vi "Create Lookup Table Envelope Waveform.vi"(0 "Reference Waveform":T2 {"Runtime Scaling" format="%#_6p"; "Sample Rate" format="%#_6p"; "Burst Length (s)" format="%#_6p"; "PAPR (dB)" format="%.2f"; "Signal Bandwidth (Hz)" format="%#_6p"}, 5 "Lookup Table Configuration":T1={"DUT Average Input Power (dBm)"=0.0, "DUT Input Power (dBm)"=array[1024 elements], "Supply Voltage (V)"=array[1024 elements]}, 11 "error in (no error)":errorcluster) -> (4 "Lookup Table Envelope Waveform":T2 {"Runtime Scaling" format="%#_6p"; "Sample Rate" format="%#_6p"; "Burst Length (s)" format="%#_6p"; "PAPR (dB)" format="%.2f"; "Signal Bandwidth (Hz)" format="%#_6p"}, 15 "error out":errorcluster)   [LabVIEW 2019, in "Envelope Tracking.lvlib"]
doc: "Creates an envelope waveform utilizing the lookup table method."
uses:
  Envelope Tracking.lvlib
  Common/Waveform.ctl
  Typedefs/Lookup Table Configuration.ctl
  <vilib>/gmath/NI_Gmath.lvlib
  Common/Common.lvlib
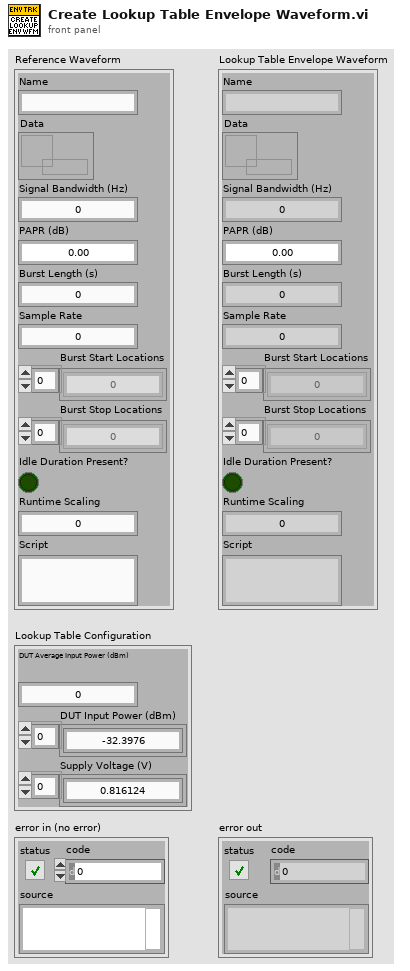
[diagram p1: front panel]
types:
  T1 = typedef "Envelope Tracking.lvlib/Lookup Table Configuration.ctl" = cluster{"DUT Average Input Power (dBm)":dbl, "DUT Input Power (dBm)":sgl[], "Supply Voltage (V)":sgl[]}
  T2 = typedef "Common.lvlib/Waveform.ctl" = cluster{"Name":string, "Data":refnum<data-value>, "Signal Bandwidth (Hz)":dbl, "PAPR (dB)":dbl, "Burst Length (s)":dbl, "Sample Rate":dbl, "Burst Start Locations":i32[], "Burst Stop Locations":i32[], "Idle Duration Present?":bool, "Runtime Scaling":dbl, "Script":string}
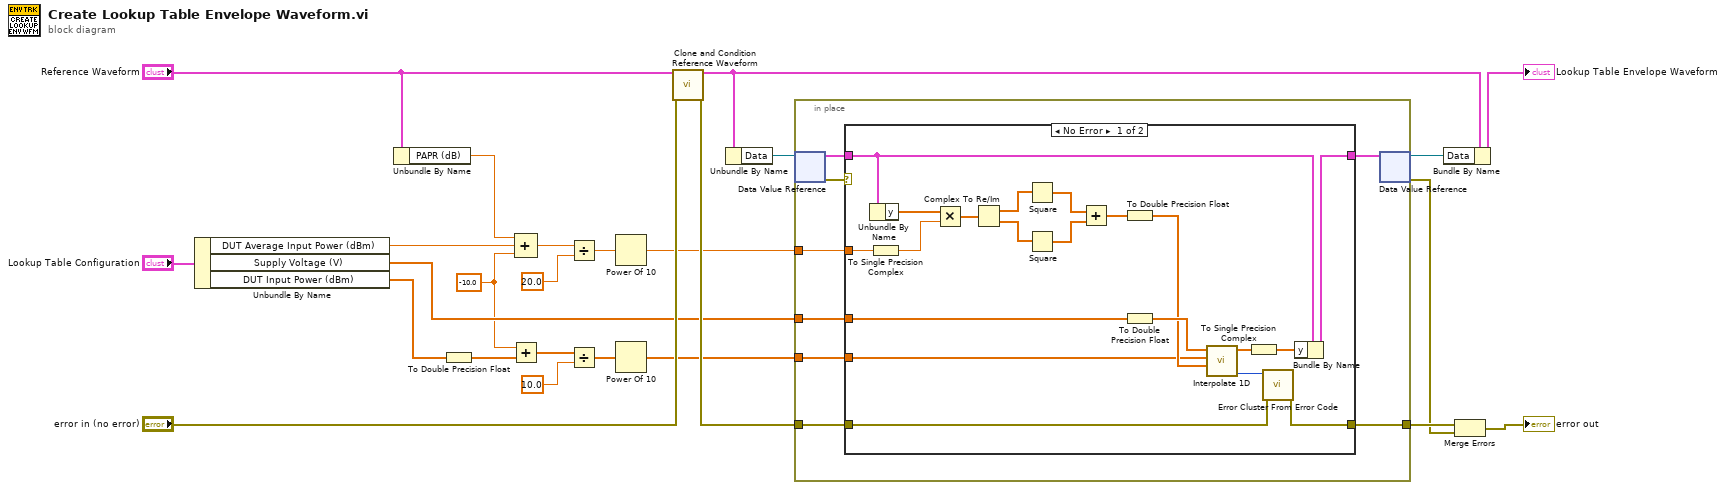
[diagram p0: block diagram]
diagram:
  w12 = -10.0 ("value")
  n1 = Unbundle By Name("Lookup Table Configuration") -> ("DUT Average Input Power (dBm)"=w19:dbl, "Supply Voltage (V)"=w14:sgl[], "DUT Input Power (dBm)"=w13:sgl[])
  n2 = Unbundle By Name("Reference Waveform") -> ("PAPR (dB)"=w1:dbl)
  n3 = To Double Precision Float(number=w13) -> (double precision float=w11:dbl[])
  n4 = Add(x=w12, y=w11) -> (x+y=w10:dbl[])
  n5 = Compound Arithmetic op=ADD(w1, w19, w12) -> (w18:dbl)
  n6 = Divide(x=w18, y=20.0) -> (x/y=w16:dbl)
  n7 = Divide(x=w10, y=10.0) -> (x/y=w8:dbl[])
  n8 = Power Of 10(x=w16) -> (10^x=w15:dbl)
  n9 = Power Of 10(x=w8) -> (10^x=w7:dbl[])
  n10 = call "Clone and Condition Reference Waveform.vi"("Reference Waveform"="Reference Waveform", "error in (no error)"="error in (no error)") -> ("Conditioned Reference Waveform"=w5:T2, "error out"=w24:errorcluster)  [unwired: 12 in]
  n11 = Unbundle By Name(w5) -> ("Data"=w4:refnum<data-value>)
  n12 = in-place {
    in-place-border: [w32] -> w23
    in-place-border: w15 -> [w30]
    in-place-border: w14 -> [w29]
    in-place-border: w7 -> [w28]
    in-place-border: w24 -> [w33]
    n13 = in-place-dvr #1(w4) -> (w27:cluster{"t0":dbl, "dt":dbl, "y":csg[]}, w31:errorcluster)
    n14 = case shown="No Error" w31 {
      tunnel: w30 -> [w51 _]
      tunnel: w29 -> [w43 _]
      tunnel: w28 -> [w39 _]
      tunnel: w27 -> [w35 w54]
      tunnel: w33 -> [w53 w55]
      tunnel: [w34 w54] -> w26
      tunnel: [w52 w55] -> w32
      frame No Error {
        n15 = Unbundle By Name(w35) -> ("y"=w49:csg[])
        n16 = To Single Precision Complex(1:w51) -> (0:w50:csg)
        n17 = Multiply(x=w49, y=w50) -> (x*y=w48:csg[])
        n18 = Complex To Re/Im(x + iy=w48) -> (x=w47:sgl[], y=w46:sgl[])
        n19 = Square(x=w47) -> (x^2=w45:sgl[])
        n20 = Square(x=w46) -> (x^2=w44:sgl[])
        n21 = Add(x=w45, y=w44) -> (x+y=w41:sgl[])
        n22 = To Double Precision Float(number=w41) -> (double precision float=w40:dbl[])
        n23 = To Double Precision Float(number=w43) -> (double precision float=w42:dbl[])
        n24 = call <vilib>:"Interpolate 1D.vi"("xi"=w40, "X"=w39, "Y"=w42) -> ("error"=w38:i32, "yi"=w37:dbl[])  [unwired: 6 in, 1 out]
        n25 = To Single Precision Complex(1:w37) -> (0:w36:csg[])
        n26 = call <vilib>:"Error Cluster From Error Code.vi"("error in (no error)"=w53, "error code (0)"=w38) -> ("error out"=w52:errorcluster)  [unwired: 7 in]
        n27 = Bundle By Name(cluster=w35, "y"=w36) -> (w34:cluster{"t0":dbl, "dt":dbl, "y":csg[]})
      }
      frame Error {
      }
    }
    n28 = in-place-dvr #1(w26) -> (w3:refnum<data-value>, w22:errorcluster)
  }
  n29 = Bundle By Name(cluster=w5, "Data"=w3) -> (→"Lookup Table Envelope Waveform":T2)
  n30 = Merge Errors(w23, w22) -> (→"error out":errorcluster)
